vi "Record Filename.vi"(8 "error in (no error)":errorcluster, 10 "Filename":string, 11 "VISA resource name":refnum<visa-resource-name>) -> (0 "error out":errorcluster, 3 "VISA resource name out":refnum<visa-resource-name>)   [LabVIEW 2017, in "Sefram DAS220.lvlib"]
doc: "Set the record filename."
uses:
  <instrlib>/Sefram DAS220/Sefram DAS220.lvlib
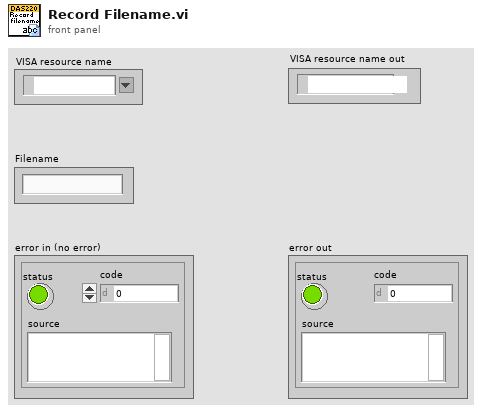
[diagram p1: front panel]
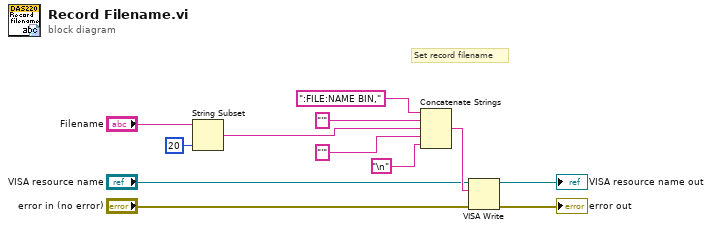
[diagram p0: block diagram]
diagram:
  # "Set record filename"
  n1 = String Subset(string="Filename", length (rest)=20 ("length (rest)")) -> (substring=w2:string)  [unwired: 1 in]
  n2 = Concatenate Strings(":FILE:NAME BIN," ("string"), "'" ("string"), w2, "'" ("string"), "\n") -> (w12:string)
  n3 = VISA Write(VISA resource name="VISA resource name", write buffer=w12, error in (no error)="error in (no error)") -> (VISA resource name out=→"VISA resource name out":refnum<visa-resource-name>, error out=→"error out":errorcluster)  [unwired: 1 out]
